vi "Auton-PassiveCan.vi"() -> (2 "Done":bool)   [LabVIEW 2014]
uses:
  Robot Global Data.vi
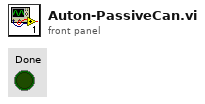
[diagram p1: front panel]
types:
  T1 = cluster{"Tote Constant":dbl, "Can2Catch Constant":dbl, "Bottom":dbl}
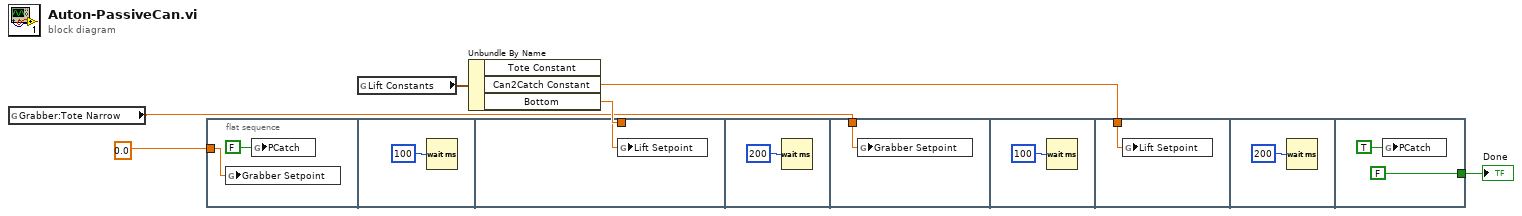
[diagram p0: block diagram]
diagram:
  n1 = global read "Robot Global Data.vi" "Grabber:Tote Narrow"() -> (w1:dbl)
  n2 = flat-sequence {
    tunnel: 0.0 -> [w7]
    tunnel: w5 -> [w10]
    tunnel: w1 -> [w12]
    tunnel: w4 -> [w14]
    tunnel: [FALSE] -> w3
    frame #0 {
      n3 = global write "Robot Global Data.vi" "Grabber Setpoint"(w7) -> ()
      n4 = global write "Robot Global Data.vi" "PCatch"(FALSE) -> ()
    }
    frame #1 {
      n5 = Wait (ms)(milliseconds to wait=u32 100) -> ()  [unwired: 1 out]
    }
    frame #2 {
      n6 = global write "Robot Global Data.vi" "Lift Setpoint"(w10) -> ()
    }
    frame #3 {
      n7 = Wait (ms)(milliseconds to wait=u32 200) -> ()  [unwired: 1 out]
    }
    frame #4 {
      n8 = global write "Robot Global Data.vi" "Grabber Setpoint"(w12) -> ()
    }
    frame #5 {
      n9 = Wait (ms)(milliseconds to wait=u32 100) -> ()  [unwired: 1 out]
    }
    frame #6 {
      n10 = global write "Robot Global Data.vi" "Lift Setpoint"(w14) -> ()
    }
    frame #7 {
      n11 = Wait (ms)(milliseconds to wait=u32 200) -> ()  [unwired: 1 out]
    }
    frame #8 {
      n12 = global write "Robot Global Data.vi" "PCatch"(TRUE ("PCatch")) -> ()
    }
  }
  n13 = global read "Robot Global Data.vi" "Lift Constants"() -> (w6:T1)
  n14 = Unbundle By Name(w6) -> ("Can2Catch Constant"=w4:dbl, "Bottom"=w5:dbl)  [unwired: 1 out]
  "Done" <- w3
